vi "Zero Sensor.vi"(7 "Channel (0: Channel A)":u16(ring) items=["Channel A", "Channel B"], 8 "error in (no error)":errorcluster, 10 "Maximum Time (120 seconds)":i16=120 min=0, 11 "BH Druck PACE Series in":refnum<class "BH Druck PACE Series.lvclass">) -> (0 "error out":errorcluster, 3 "BH Druck PACE Series out":refnum<class "BH Druck PACE Series.lvclass">)   [LabVIEW 2022 SP3, in "BH Druck PACE Series.lvclass"]
uses:
  BH Druck PACE Series.lvclass
  BH Druck PACE Series.lvclass/BH Druck PACE Series.ctl
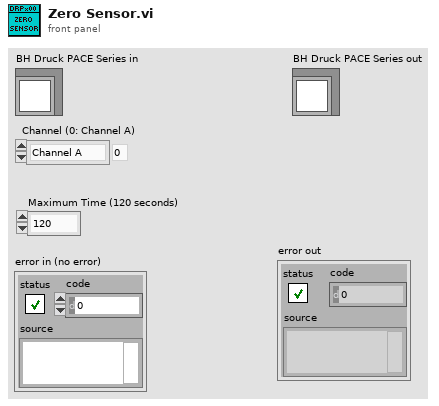
[diagram p1: front panel]
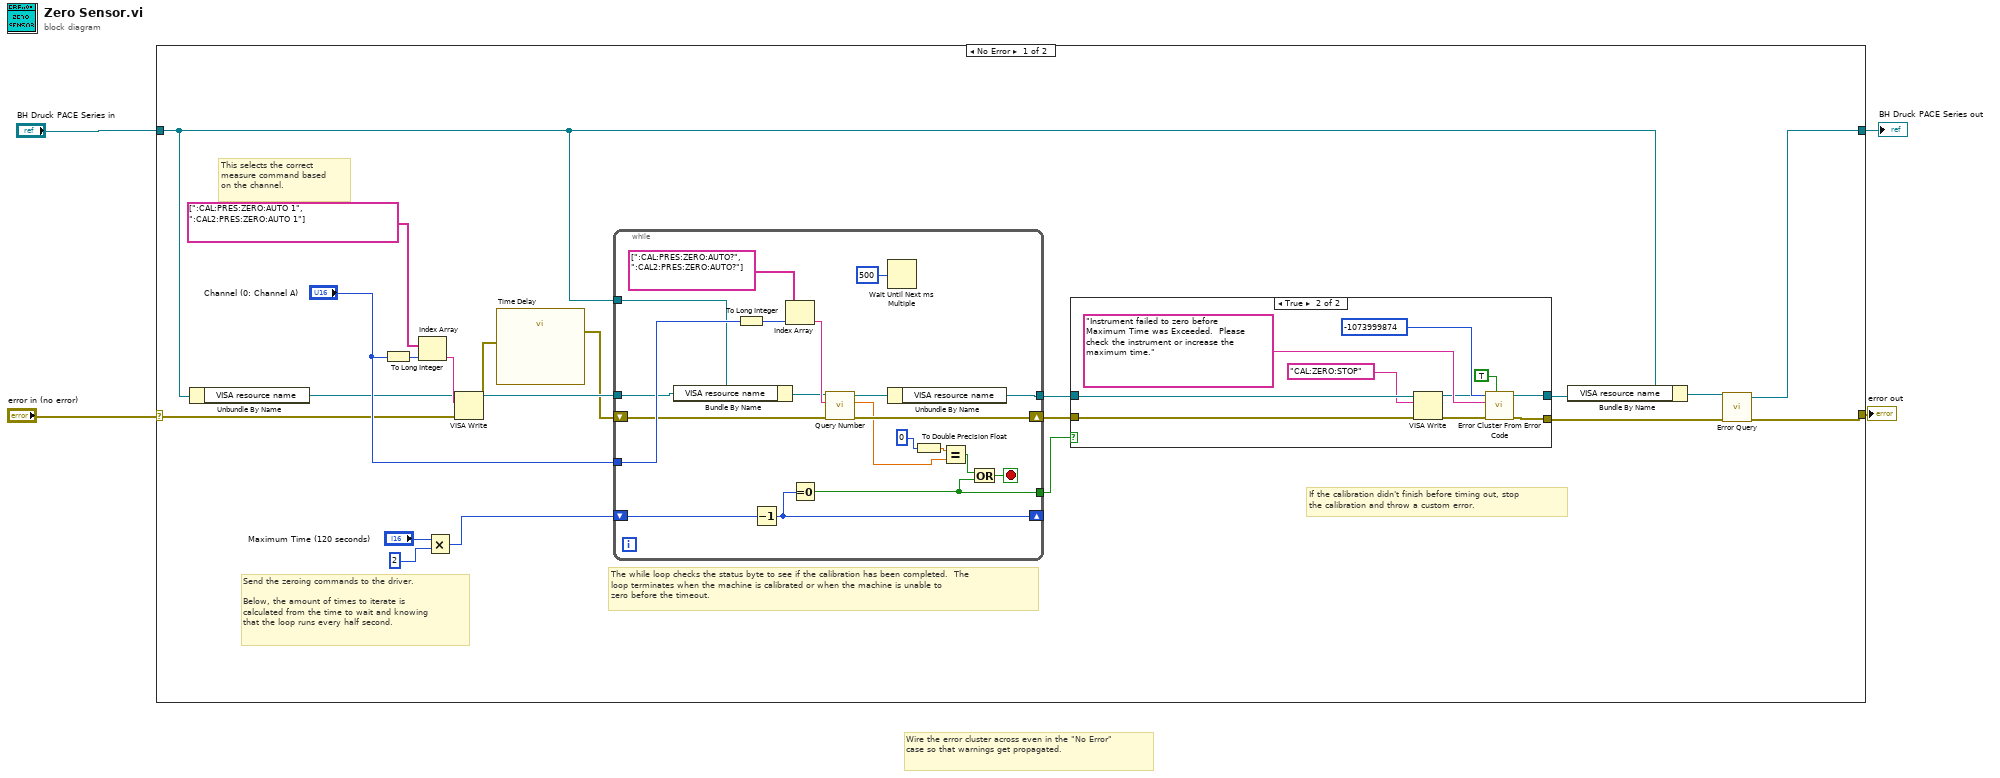
[diagram p0: block diagram]
diagram:
  # "Wire the error cluster across even in the \"No Error\"\ncase so that warnings get propagated."
  n1 = case shown="No Error" "error in (no error)" {
    selector: "error in (no error)" -> [w12 w58]
    tunnel: [w5 w58] -> w3
    tunnel: [w6 w57] -> w1
    tunnel: "BH Druck PACE Series in" -> [w9 w57]
    frame No Error {
      # "This selects the correct\nmeasure command based\non the channel."
      # "If the calibration didn't finish before timing out, stop\nthe calibration and throw a custom error."
      # "The while loop checks the status byte to see if the calibration has been completed.  The\nloop terminates when the machine is calibrated or when the machine is unable to\nzero before the timeout."
      # "Send the zeroing commands to the driver.\n\nBelow, the amount of times to iterate is\ncalculated from the time to wait and knowing\nthat the loop runs every half second."
      n2 = Unbundle By Name(w9) -> ("VISA resource name"=w11:refnum<visa-resource-name>)
      n3 = To Long Integer(number="Channel (0: Channel A)") -> (32bit integer=w10:i32)
      n4 = Index Array(array=string[] [":CAL:PRES:ZERO:AUTO 1", ":CAL2:PRES:ZERO:AUTO 1"], index=w10) -> (element=w16:string)
      n5 = Multiply(x="Maximum Time (120 seconds)", y=i16 2) -> (x*y=w22:i16)
      n6 = VISA Write(VISA resource name=w11, write buffer=w16, error in (no error)=w12) -> (VISA resource name out=w25:refnum<visa-resource-name>, error out=w14:errorcluster)  [unwired: 1 out]
      n7 = call "Time Delay"("error in (no error)"=w14) -> ("error out"=w13:errorcluster)  [unwired: 10 in]
      n8 = while {
        tunnel: w25 -> [w41]
        shift-right: [w46] -> w19
        shift-left: w13 -> [w47]
        tunnel: [w37] -> w20
        tunnel: [w52] -> w21
        shift-right: [w51] -> _
        shift-left: w22 -> [w55]
        tunnel: "Channel (0: Channel A)" -> [w48]
        tunnel: w9 -> [w42]
        stop <- w53 stop-if-true
        n9 = Bundle By Name(cluster=w42, "VISA resource name"=w41) -> (w40:refnum<class "BH Druck PACE Series.lvclass">)
        n10 = To Long Integer(number=w48) -> (32bit integer=w43:i32)
        n11 = Decrement(x=w55) -> (x-1=w51:i16)
        n12 = Index Array(array=string[] [":CAL:PRES:ZERO:AUTO?", ":CAL2:PRES:ZERO:AUTO?"], index=w43) -> (element=w45:string)
        n13 = Equal To 0?(x=w51) -> (x = 0?=w52:bool)
        n14 = call-dynamic "Query Number.vi"("error in (no error)"=w47, "Query String"=w45, "BH Druck PACE Series in"=w40) -> ("error out"=w46:errorcluster, "Numeric Result"=w44:dbl, "BH Druck PACE Series out"=w38:refnum<class "BH Druck PACE Series.lvclass">)  [unwired: 6 in]
        n15 = Wait Until Next ms Multiple(millisecond multiple=u32 500) -> ()  [unwired: 1 out]
        n16 = Unbundle By Name(w38) -> ("VISA resource name"=w37:refnum<visa-resource-name>)
        n17 = To Double Precision Float(number=i8 0 ("y")) -> (double precision float=w39:dbl)
        n18 = Equal?(x=w39, y=w44) -> (x = y?=w54:bool)
        n19 = Or(x=w54, y=w52) -> (x .or. y?=w53:bool)
      }
      n20 = case shown="True" w21 {
        tunnel: w20 -> [w27 w36]
        tunnel: w19 -> [w26 w35]
        tunnel: [w27 w29] -> w8
        tunnel: [w26 w28] -> w18
        frame False {
        }
        frame True {
          n21 = VISA Write(VISA resource name=w36, write buffer="CAL:ZERO:STOP", error in (no error)=w35) -> (VISA resource name out=w29:refnum<visa-resource-name>, error out=w30:errorcluster)  [unwired: 1 out]
          n22 = call <vilib>:"Error Cluster From Error Code.vi"("show call chain? (False)"=TRUE, "error in (no error)"=w30, "error message (\"\")"="Instrument failed to zero before Maximum Time was Exceeded.  Please check the instrument or increase the maximum time." ("error message (\"\")"), "error code (0)"=-1073999874) -> ("error out"=w28:errorcluster)  [unwired: 5 in]
        }
      }
      n23 = Bundle By Name(cluster=w9, "VISA resource name"=w8) -> (w7:refnum<class "BH Druck PACE Series.lvclass">)
      n24 = call-dynamic "Error Query.vi"("error in (no error)"=w18, "BH Druck PACE Series in"=w7) -> ("error out"=w5:errorcluster, "BH Druck PACE Series out"=w6:refnum<class "BH Druck PACE Series.lvclass">)  [unwired: 8 in]
    }
    frame Error {
    }
  }
  "error out" <- w3
  "BH Druck PACE Series out" <- w1
